vi "main.vi"() -> ()   [LabVIEW 2017, in "模块B.lvlib"]
panel:
  in  "B":dbl=100.0 format="%#_13g"
  out "数值":dbl
  out "字符串":string
  # "B"
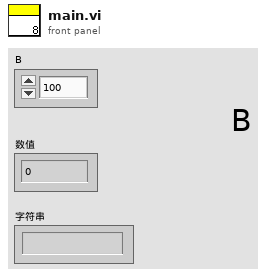
[diagram p1: front panel]
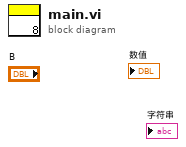
[diagram p0: block diagram]
diagram:
